vi "disconnect.vi"(8 "error in (no error)":errorcluster, 11 "CoolerControler in":refnum<class "CoolerControler.lvclass">) -> (0 "error out":errorcluster, 3 "CoolerControler out":refnum<class "CoolerControler.lvclass">)   [LabVIEW 2016, in "CoolerControler.lvclass"]
uses:
  CoolerControler.lvclass
  CoolerControler.lvclass/CoolerControler.ctl
  common_serial_tcpextended/Communicator/Communicator.lvclass
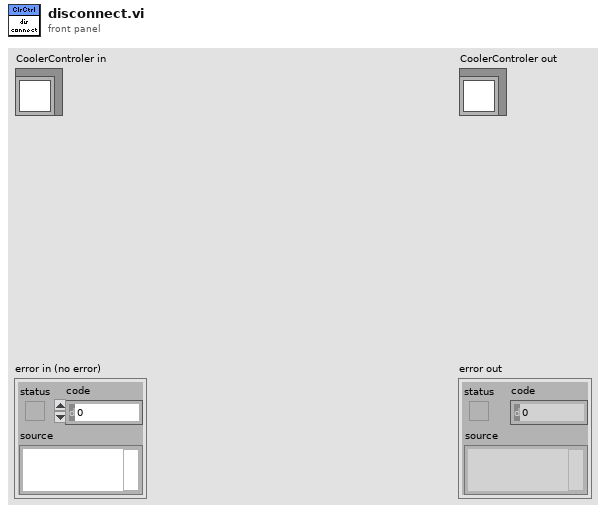
[diagram p1: front panel]
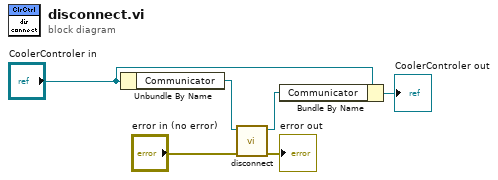
[diagram p0: block diagram]
diagram:
  n1 = Unbundle By Name("CoolerControler in") -> ("Communicator"=w4:refnum<class "Communicator.lvclass">)
  n2 = call-dynamic "disconnect.vi"("error in (no error)"="error in (no error)", "Communicator in"=w4) -> ("error out"=→"error out":errorcluster, "Communicator out"=w3:refnum<class "Communicator.lvclass">)  [unwired: 8 in]
  n3 = Bundle By Name(cluster="CoolerControler in", "Communicator"=w3) -> (→"CoolerControler out":refnum<class "CoolerControler.lvclass">)
